vi "Hex Str to U8 Data.vi"(1 "HEX String (0-9,A-F)":string) -> (0 "U8 Data[]":u8[](array[numeric]) format="%.0x")   [LabVIEW 2017, in "Communicable State Machine.lvlib"]
doc: "### Hex Str to U8 Data.vi\n\n-- <b>Controls</b> --\n- <b>HEX String (0-9,A-F)</b>:\n\n-- <b>Indicators</b> --\n- <b>u8 Data[]</b>:"
uses:
  Communicable State Machine.lvlib
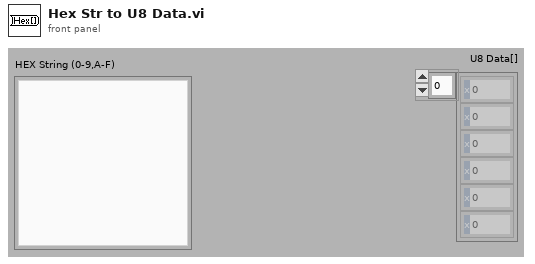
[diagram p1: front panel]
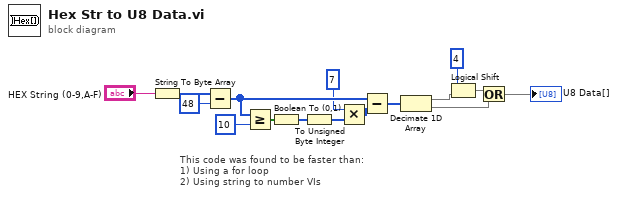
[diagram p0: block diagram]
diagram:
  # "This code was found to be faster than:\n1) Using a for loop\n2) Using string to number VIs"
  n1 = String To Byte Array(string="HEX String (0-9,A-F)") -> (unsigned byte array=w1:u8[])
  n2 = Subtract(x=w1, y=u8 48) -> (x-y=w14:u8[])
  n3 = Greater Or Equal?(x=w14, y=u8 10) -> (x >= y?=w11:bool[])
  n4 = Boolean To (0,1)(Boolean=w11) -> (0, 1=w9:i16[])
  n5 = To Unsigned Byte Integer(number=w9) -> (unsigned 8bit integer=w12:u8[])
  n6 = Multiply(x=u8 7, y=w12) -> (x*y=w13:u8[])
  n7 = Subtract(x=w14, y=w13) -> (x-y=w3:u8[])
  n8 = Decimate 1D Array(w3) -> (w4:u8[], w2:u8[])
  n9 = Logical Shift(y=i8 4, x=w4) -> (x << y=w15:u8[])
  n10 = Or(x=w15, y=w2) -> (x .or. y?=→"U8 Data[]":u8[])
